vi "Write TogglePower Event.vi"(8 "error in":errorcluster, 10 "TogglePower Event":refnum<user-event>, 11 "Engine in":refnum<class "Engine.lvclass">) -> (0 "error out":errorcluster, 3 "Engine out":refnum<class "Engine.lvclass">)   [LabVIEW 2019, in "Engine.lvlib" / "Engine.lvclass"]
uses:
  Project/Engine.lvclass
  Project/Engine.lvclass/Engine.ctl
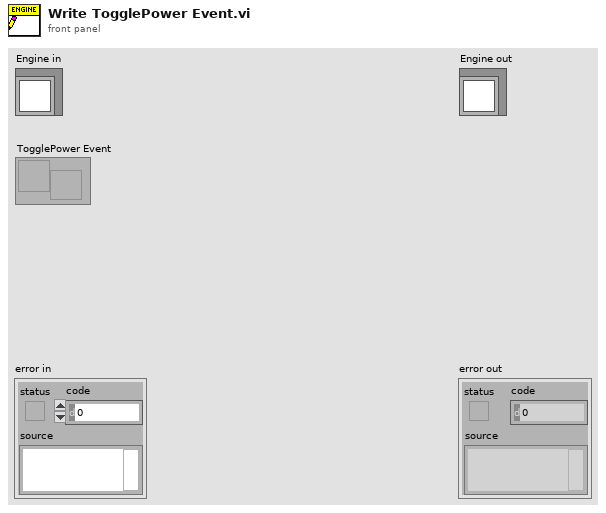
[diagram p1: front panel]
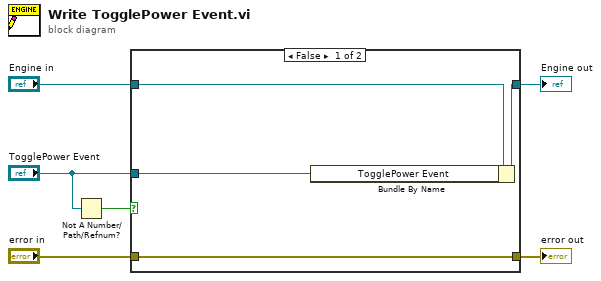
[diagram p0: block diagram]
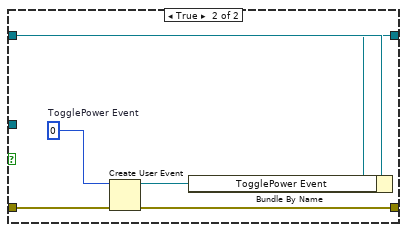
[diagram p2: hidden frame]
diagram:
  n1 = Not A Number/Path/Refnum?(number/path/refnum="TogglePower Event") -> (NaN/Path/Refnum?=w3:bool)
  n2 = case shown="False" w3 {
    tunnel: [w7 w13] -> w1
    tunnel: [w9 w12] -> w5
    tunnel: "Engine in" -> [w10 w16]
    tunnel: "TogglePower Event" -> [w8 _]
    tunnel: "error in" -> [w7 w14]
    frame False {
      n3 = Bundle By Name(cluster=w10, "TogglePower Event"=w8) -> (w9:refnum<class "Engine.lvclass">)
    }
    frame True {
      w15 = 0  # TogglePower Event
      n4 = Create User Event(user event datatype=w15, error in=w14) -> (user event=w11:refnum<user-event>, error out=w13:errorcluster)
      n5 = Bundle By Name(cluster=w16, "TogglePower Event"=w11) -> (w12:refnum<class "Engine.lvclass">)
    }
  }
  "error out" <- w1
  "Engine out" <- w5
